vi "Label_bottles.vi"() -> (0 "Array":T1(array[cluster]))   [LabVIEW 2016]
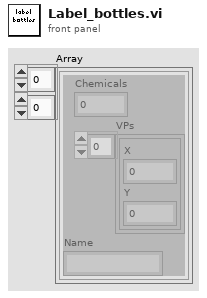
[diagram p1: front panel]
types:
  T1 = cluster{"Chemicals":i32, "VPs":cluster{"X":dbl, "Y":dbl}[], "Name":string}[][]
  T2 = cluster{"Chemicals":i32, "VPs":cluster{"X":dbl, "Y":dbl}[], "Name":string}
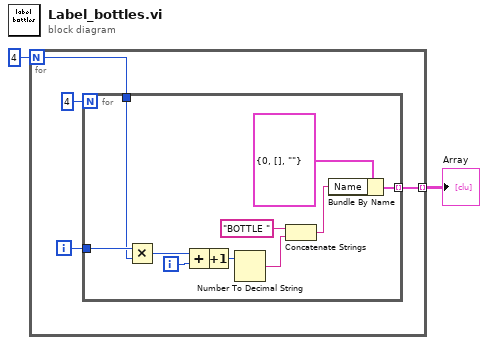
[diagram p0: block diagram]
diagram:
  n1 = for {
    N: 4 -> [w4]
    tunnel: [w6] -> w1 mode=indexing
    i -> [w5]
    n2 = for {
      N: 4 -> [_]
      tunnel: [w17] -> w6 mode=indexing
      tunnel: w5 -> [w15]
      tunnel: w4 -> [w7]
      i -> [w13]
      n3 = Multiply(x=w15, y=w7) -> (x*y=w14:i32)
      n4 = Add(x=w14, y=w13) -> (x+y=w12:i32)
      n5 = Increment(x=w12) -> (x+1=w8:i32)
      n6 = Number To Decimal String(number=w8) -> (decimal integer string=w11:string)  [unwired: 1 in]
      n7 = Concatenate Strings("BOTTLE " ("string"), w11) -> (w9:string)
      n8 = Bundle By Name(cluster=T2 {"Chemicals"=0, "VPs"=[], "Name"=""} ("Bottle"), "Name"=w9) -> (w17:T2)
    }
  }
  "Array" <- w1
